vi "Build Spec Engine.vi"(8 "error in (no error)":errorcluster, 9 "Action":T1) -> (0 "error out":errorcluster, 1 "Output":string)   [LabVIEW 2014, in "CD model script.lvlib"]
doc: "Constants, which are necessary for the <B>CD Engine LLB</B> in the generated custom device."
uses:
  CD model script.lvlib
  Constants TypDef/Build Spec Engine.ctl
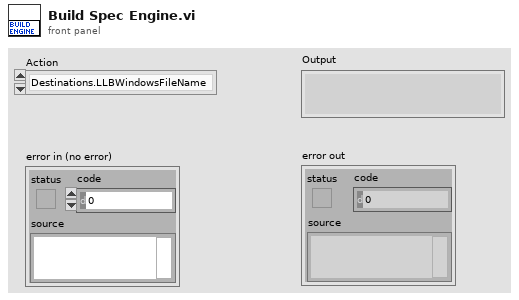
[diagram p1: front panel]
types:
  T1 = typedef "CD model script.lvlib/Build Spec Engine.ctl" = enum16{"Destinations.LLBWindowsFileName", "Destinations.LLBVxWorksFileName", "Destinations.LLBPharlapFileName", "Destinations.LLBLinuxARMFileName", "Destinations.LLBLinux64FileName"}
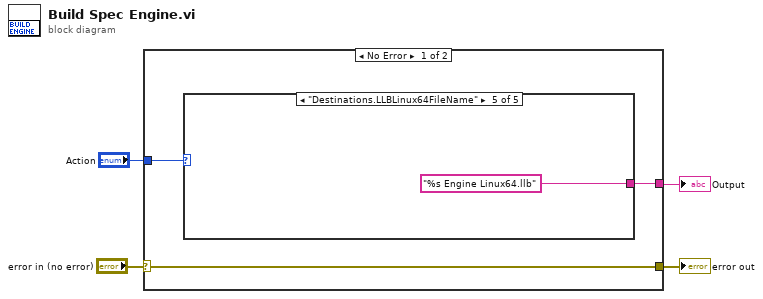
[diagram p0: block diagram]
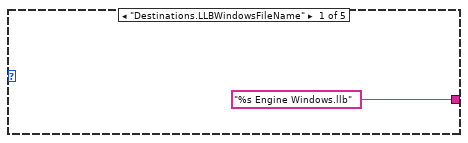
[diagram p2: hidden frame]
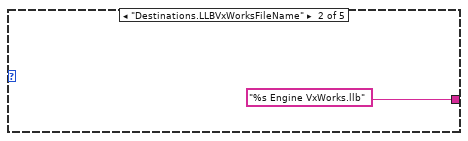
[diagram p3: hidden frame]
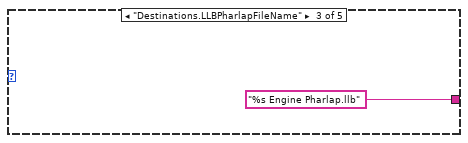
[diagram p4: hidden frame]
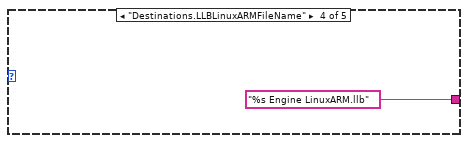
[diagram p5: hidden frame]
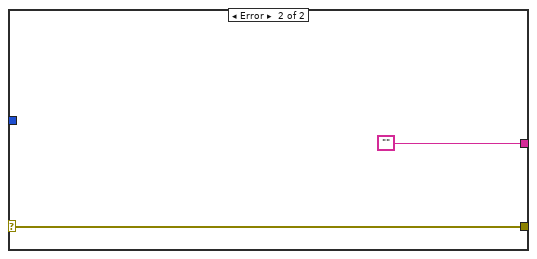
[diagram p6: hidden frame]
diagram:
  n1 = case shown="No Error" "error in (no error)" {
    selector: "error in (no error)" -> [w7 w14]
    tunnel: [w7 w14] -> w3
    tunnel: [w5 ""] -> w2
    tunnel: "Action" -> [w6 _]
    frame No Error {
      n2 = case shown="\"Destinations.LLBLinux64FileName\"" w6 {
        tunnel: ["%s Engine Windows.llb" "%s Engine VxWorks.llb" "%s Engine Pharlap.llb" "%s Engine LinuxARM.llb" "%s Engine Linux64.llb"] -> w5
        frame "Destinations.LLBWindowsFileName" {
        }
        frame "Destinations.LLBVxWorksFileName" {
        }
        frame "Destinations.LLBPharlapFileName" {
        }
        frame "Destinations.LLBLinuxARMFileName" {
        }
        frame "Destinations.LLBLinux64FileName" {
        }
      }
    }
    frame Error {
    }
  }
  "error out" <- w3
  "Output" <- w2
